vi "Position et T max.vi"() -> ()   [LabVIEW 2018]
panel:
  out "Data Out":dbl[](array[numeric])
  in  "DATA In":dbl[](array[numeric])
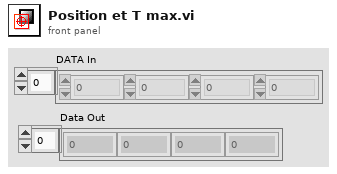
[diagram p1: front panel]
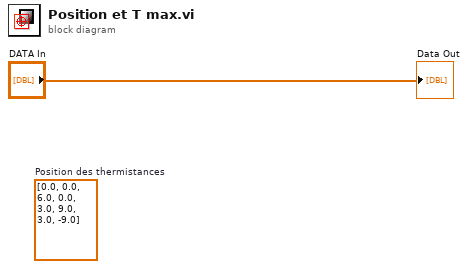
[diagram p0: block diagram]
diagram:
  (unwired) dbl[][] [[0.0, 0.0], [6.0, 0.0], [3.0, 9.0], [3.0, -9.0]]  # Position des thermistances
  "Data Out" <- "DATA In"
